vi "ConstantToArray_U32Color.vi"(11 "Constant":u32) -> (3 "ConstantArray":dbl[](array[numeric]))   [LabVIEW 2020, in "OpenLvVision_OpenCv.lvlib"]
uses:
  OpenLvVision_OpenCv.lvlib
  <vilib>/OpenLvVision/OpenLvVision_Image/DataAccess/OLV DataAccess.lvlib
  <vilib>/OpenLvVision/OpenLvVision_Image/DataAccess/NumberToColor/OLV U32toRgba.vi
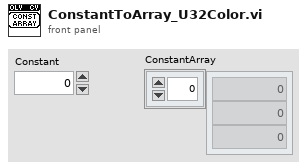
[diagram p1: front panel]
types:
  T1 = typedef "OLV OpenLvVision_Image.lvlib/OLV DataAccess.lvlib/OLV RgbaU32.ctl" = cluster{"Plane 1 (Red)":u8, "Plane 2 (Green)":u8, "Plane 3 (Blue)":u8, "Plane 4 (alpha)":u8}
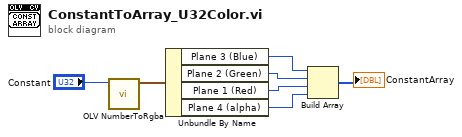
[diagram p0: block diagram]
diagram:
  n1 = call-poly <vilib>:"OLV NumberToRgba.vi"("U32"="Constant") -> ("Rgba"=w6:T1)  [unwired: 10 in]
  n2 = Unbundle By Name(w6) -> ("Plane 3 (Blue)"=w5:u8, "Plane 2 (Green)"=w4:u8, "Plane 1 (Red)"=w3:u8, "Plane 4 (alpha)"=w2:u8)
  n3 = Build Array(w5, w4, w3, w2) -> (→"ConstantArray":u8[])
